vi "Main.vi"() -> ()   [LabVIEW 2014]
doc: "This example re-implements the official Dual Mode Thermometer XControl example using LQ.\n\nFor the best results, study this project alongside \"Simple Dual Mode Thermometer XControl.lvproj\".\n\n Go to \"Help\" -> \"Find Examples...\" -> \"Search\". Enter the keywords: \"Simple Dual Mode Thermometer\".\n\n<b>Similarities with XControls</b>\n* Widgets and XControls are reusable user-created GUI components.\n* Widgets and XControls support Property Nodes.\n\n<b>Differences from XControls</b>\n* You can inherit from a Widget.\n* Widgets (and LVOOP) don't support invoke nodes (as of LabVIEW 2018). Call the associated VI directly.\n* While XControls have separate Data and State abilities, Widgets don't make this distinction.\n * While XControls use block diagram terminals, Widgets use Property Nodes or VIs.\n* While XControls have separate Facade and Init VIs, Widgets handle both of these in their Constructor VI.\n\n\nCopyright (c) 2019 Sze Howe Koh.\nThis code is licensed under the MIT license."
uses:
  <vilib>/addons/LQ/Qt Widgets/LQWidgetEngine/LQWidgetEngine.lvclass
  Dual Mode Thermometer/Get Temperature (Celsius).vi
  Dual Mode Thermometer/Set Temperature (Celsius).vi
  Dual Mode Thermometer/Is Farenheit Mode.vi
  <vilib>/addons/LQ/LQ Core/LQCoreEngine/LQCoreEngine.lvclass
  Dual Mode Thermometer/Dual Mode Thermometer.lvclass
panel:
  out "Degrees Fahrenheit":dbl
  in  "Degrees Celsius":dbl
  out "Farenheit?":bool
  in  "Stop Button":bool
  # "Overview: This VI demonstrates the functionality of the Dual Mode Thermometer Widget.\nInstructions:\n1. Run the VI.\n2. Adjust the DMTC.\n3. Select the Fahrenheit mode of DMTC.\n4. Adjust the DMTC.\n5. Select the Fahrenheit mode of DMTI.\n6. Adjust the DMTC.\n7. Click Stop to stop the VI.\n\nNote: Unlike XControls, you don't need to close this VI before making any changes to the Dual Mode Thermometer Widget."
  # "For the best results, study this project alongside \"Simple Dual Mode Thermometer XControl.lvproj\".\n\n        Go to \"Help\" -> \"Find Examples...\" -> \"Search\". Enter the keywords: \"Simple Dual Mode Thermometer\".\n\nSimilarities with XControls\n* Widgets and XControls are reusable user-created GUI components.\n* Widgets and XControls support Property Nodes.\n\nDifferences from XControls\n* You can inherit from a Widget.\n* Widgets (and LVOOP) don't support invoke nodes (as of LabVIEW 2018). Call the associated VI directly.\n* While XControls have separate Data and State abilities, Widgets don't make this distinction.\n        * While XControls use block diagram terminals, Widgets use Property Nodes or VIs.\n* While XControls have separate Facade and Init VIs, Widgets handle both of these in their Constructor VI."
  # "Temperature Converter"
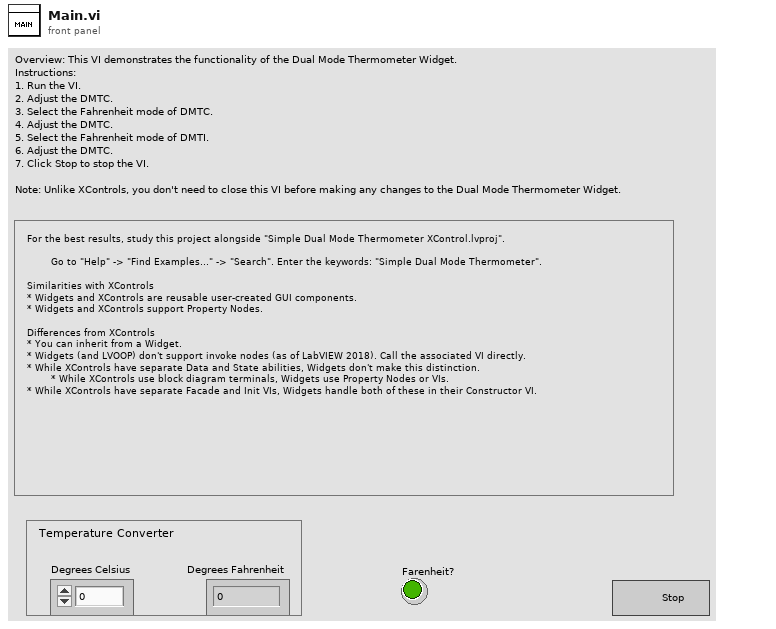
[diagram p1: front panel]
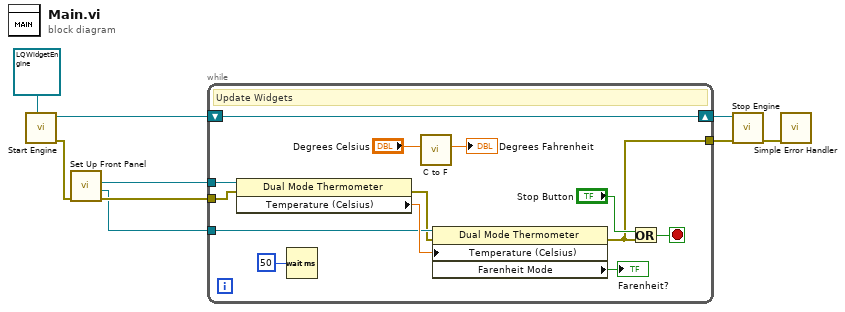
[diagram p0: block diagram]
diagram:
  n1 = call <vilib>:"Start Engine.vi"("Engine Type"=refnum<class "LQWidgetEngine.lvclass"> refnum ("Qt Widgets.lvlib:LQWidgetEngine")) -> ("Error Out"=w5:errorcluster, "New Engine"=w8:refnum<class "LQWidgetEngine.lvclass">)  [unwired: 9 in]
  n2 = call "Set Up Front Panel.vi"("Error In"=w5) -> ("Error Out"=w4:errorcluster, "Dual Mode Thermometer Indicator"=w2:refnum<class "Dual Mode Thermometer.lvclass">, "Dual Mode Thermometer Control"=w1:refnum<class "Dual Mode Thermometer.lvclass">)  [unwired: 8 in]
  n3 = while {
    shift-right: [w22] -> w7
    shift-left: w8 -> [w22]
    tunnel: w2 -> [w15]
    tunnel: [w11] -> w6
    tunnel: w1 -> [w17]
    tunnel: w4 -> [w14]
    stop <- w10 stop-if-true
    # "Update Widgets"
    n4 = property class="Dual Mode Thermometer"(reference=w17, error in=w14) -> (error out=w13:errorcluster, "Temperature (Celsius)"=w16:dbl)  [unwired: 1 out]
    n5 = Wait (ms)(milliseconds to wait=u32 50) -> ()  [unwired: 1 out]
    n6 = call "C to F.vi"("Value [°C]"="Degrees Celsius") -> ("Value [°F]"=→"Degrees Fahrenheit":dbl)  [unwired: 10 in]
    n7 = property class="Dual Mode Thermometer"(reference=w15, error in=w13, "Temperature (Celsius)"=w16) -> (error out=w11:errorcluster, "Farenheit Mode"=→"Farenheit?":bool)  [unwired: 1 out]
    n8 = Or(x="Stop Button", y=w11) -> (x .or. y?=w10:bool)
  }
  n9 = call <vilib>:"Stop Engine.vi"("Error In"=w6, "LQCoreEngine"=w7) -> ("Error Out"=w3:errorcluster)  [unwired: 9 in]
  n10 = call <vilib>:"Simple Error Handler.vi"("error in (no error)"=w3) -> ()  [unwired: 4 in, 5 out]
